vi "Write Resources.vi"(8 "error in (no error)":errorcluster, 10 "Resources []":T1[](array[typedef]), 11 "ResFile in":refnum<class "Resource Data.lvclass">) -> (0 "error out":errorcluster, 3 "ResFile out":refnum<class "Resource Data.lvclass">)   [LabVIEW 2013, in "SET Project Data.lvlib" / "Resource Data.lvclass"]
uses:
  Resource Data.lvclass
  Types/ProjFile_Resource Entry.ctl
  Resource Data.lvclass/Resource Data.ctl
  SET Project Data.lvlib
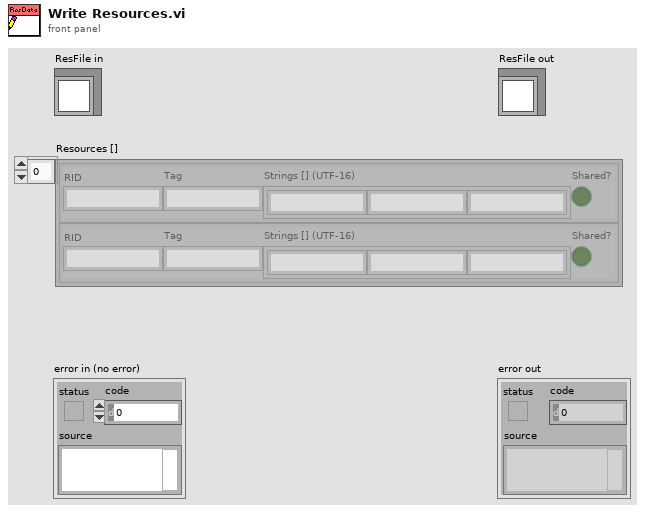
[diagram p1: front panel]
types:
  T1 = typedef "SET Project Data.lvlib/ProjFile_Resource Entry.ctl" = cluster{"RID":string, "Tag":string, "Strings [] (UTF-16)":string[], "Shared?":bool}
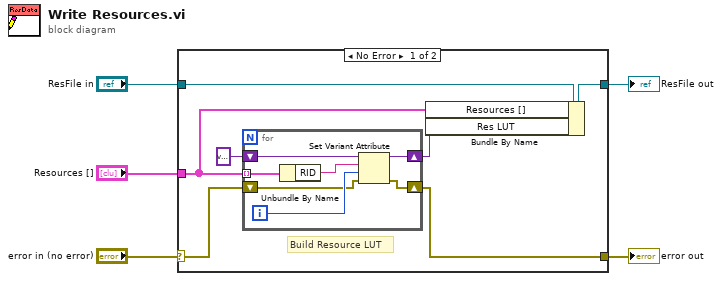
[diagram p0: block diagram]
diagram:
  n1 = case shown="No Error" "error in (no error)" {
    selector: "error in (no error)" -> [w7 w20]
    tunnel: [w6 w20] -> w4
    tunnel: [w11 w21] -> w2
    tunnel: "ResFile in" -> [w12 w21]
    tunnel: "Resources []" -> [w8 _]
    frame No Error {
      # "Build Resource LUT"
      n2 = for {
        tunnel: w8 -> [w19] mode=indexing
        shift-right: [w18] -> w9
        shift-left: variant ("variant") -> [w17]
        shift-right: [w13] -> w6
        shift-left: w7 -> [w14]
        i -> [w15]
        n3 = Unbundle By Name(w19) -> ("RID"=w16:string)
        n4 = Set Variant Attribute(Variant=w17, name=w16, value=w15, error in=w14) -> (Variant out=w18:variant, error out=w13:errorcluster)  [unwired: 1 out]
      }
      n5 = Bundle By Name(cluster=w12, "Resources []"=w8, "Res LUT"=w9) -> (w11:refnum<class "Resource Data.lvclass">)
    }
    frame Error {
    }
  }
  "error out" <- w4
  "ResFile out" <- w2
